vi "toStringArray.vi"(8 "error in (no error)":errorcluster, 11 "SingleToneRamp in":refnum<class "SingleToneRamp.lvclass">) -> (0 "error out":errorcluster, 2 "eventStringArray":string[](array[string]), 3 "SingleToneRamp out":refnum<class "SingleToneRamp.lvclass">)   [LabVIEW 2011, in "Tools.lvlib" / "Scripting.lvlib" / "SingleToneRamp.lvclass"]
uses:
  SingleToneRamp.lvclass
  SingleTone.lvclass
  SingleToneRamp.lvclass/SingleToneRamp.ctl
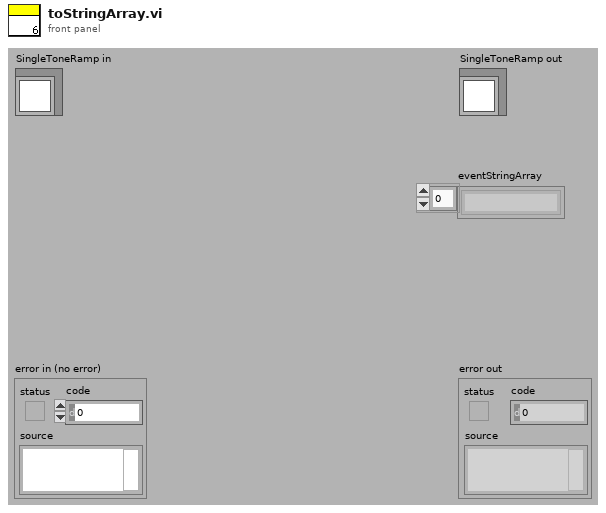
[diagram p1: front panel]
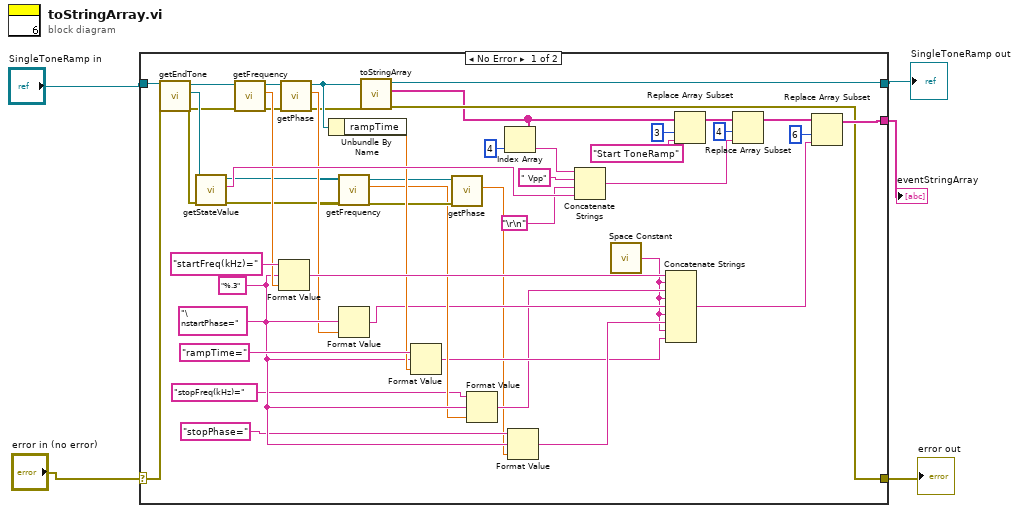
[diagram p0: block diagram]
diagram:
  n1 = case shown="No Error" "error in (no error)" {
    selector: "error in (no error)" -> [w31 w53]
    tunnel: "SingleToneRamp in" -> [w33 w54]
    tunnel: [w52 w54] -> w4
    tunnel: [w42 w53] -> w2
    tunnel: [w43 _] -> w3
    frame No Error {
      w22 = "%.3"
      n2 = call "getEndTone.vi"("error in (no error)"=w31, "SingleToneRamp.lvclass in"=w33) -> ("error out"=w17:errorcluster, "endTone"=w32:refnum<class "SingleTone.lvclass">, "SingleToneRamp.lvclass out"=w26:refnum<class "SingleToneRamp.lvclass">)  [unwired: 7 in]
      n3 = call-dynamic "getStateValue.vi"("error in (no error)"=w17, "ScriptEvent in"=w32) -> ("error out"=w18:errorcluster, "stateValue"=w35:string, "ScriptEvent out"=w19:refnum<class "SingleTone.lvclass">)  [unwired: 7 in]
      n4 = call "getFrequency.vi"("error in (no error)"=w17, "SingleTone.lvclass in"=w26) -> ("error out"=w28:errorcluster, "frequency"=w30:dbl, "SingleTone.lvclass out"=w27:refnum<class "SingleToneRamp.lvclass">)  [unwired: 7 in]
      n5 = Format Value(string ("")="startFreq(kHz)=", format string=w22, value (0)=w30) -> (output string=w45:string)
      n6 = call "getPhase.vi"("error in (no error)"=w28, "SingleTone.lvclass in"=w27) -> ("error out"=w23:errorcluster, "phase"=w24:dbl, "SingleTone.lvclass out"=w25:refnum<class "SingleToneRamp.lvclass">)  [unwired: 7 in]
      n7 = Unbundle By Name(w25) -> ("rampTime"=w29:dbl)
      n8 = call "getFrequency.vi"("error in (no error)"=w18, "SingleTone.lvclass in"=w19) -> ("error out"=w21:errorcluster, "frequency"=w16:dbl, "SingleTone.lvclass out"=w20:refnum<class "SingleTone.lvclass">)  [unwired: 7 in]
      n9 = Format Value(string ("")="\nstartPhase=", format string=w22, value (0)=w24) -> (output string=w13:string)
      n10 = call-parent "toStringArray.vi"("error in (no error)"=w23, "SingleTone in"=w25) -> ("error out"=w42:errorcluster, "eventStringArray"=w38:string[], "SingleTone out"=w52:refnum<class "SingleToneRamp.lvclass">)  [unwired: 7 in]
      n11 = Format Value(string ("")="rampTime=", format string=w22, value (0)=w29) -> (output string=w11:string)
      n12 = call "getPhase.vi"("error in (no error)"=w21, "SingleTone.lvclass in"=w20) -> ("phase"=w8:dbl)  [unwired: 7 in, 2 out]
      n13 = Format Value(string ("")="stopFreq(kHz)=", format string=w22, value (0)=w16) -> (output string=w10:string)
      n14 = Index Array(array=w38, index=4) -> (element=w36:string)
      n15 = Format Value(string ("")="stopPhase=", format string=w22, value (0)=w8) -> (output string=w12:string)
      n16 = Concatenate Strings(w36, " Vpp", "\r\n", w35) -> (w34:string)
      n17 = call <vilib>:"Space Constant.vi"() -> ("String"=w9:string)
      n18 = Concatenate Strings(w45, w9, w10, w9, w13, w9, w12, w9, w11) -> (w44:string)
      n19 = Replace Array Subset(array=w38, new element="Start ToneRamp", index=3) -> (w41:string[])
      n20 = Replace Array Subset(array=w41, new element=w34, index=4) -> (w40:string[])
      n21 = Replace Array Subset(array=w40, new element=w44, index=6) -> (w43:string[])
    }
    frame Error {
    }
  }
  "error out" <- w2
  "SingleToneRamp out" <- w4
  "eventStringArray" <- w3
